vi "Kalman_Filter_Generator.vi"(8 "error in (no error)":errorcluster, 9 "Threshold":dbl, 10 "State Variance":dbl, 11 "Measurement Variance":dbl) -> (0 "error out":errorcluster, 3 "Kalman_Filter out":refnum<class "Kalman_Filter.lvclass">)   [LabVIEW 2021, in "Kalman_Filter.lvclass"]
uses:
  Kalman_Filter.lvclass
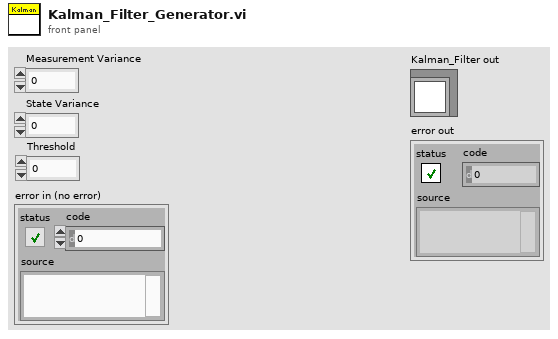
[diagram p1: front panel]
types:
  T1 = cluster{"State":dbl[][], "F state prop matrix":dbl[][], "H measure matrix":dbl[][], "P process cov":dbl[][], "R measure cov":dbl[][], "Q state cov":dbl[][], "T Sample":dbl, "New Measurement":dbl, "Measurement Variance":dbl, "State Variance":dbl, "Threshold":dbl, "Initialized":bool}
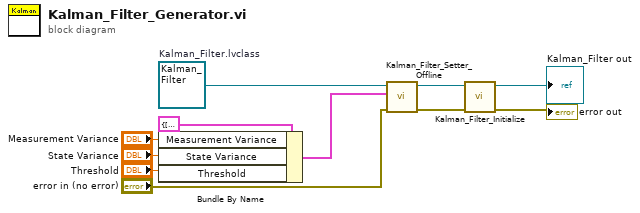
[diagram p0: block diagram]
diagram:
  w11 = refnum<class "Kalman_Filter.lvclass"> refnum  # Kalman_Filter.lvclass
  n1 = Bundle By Name(cluster=T1 {"State"=[], "F state prop matrix"=[], "H measure matrix"=[], "P process cov"=[], "R measure cov"=[], "Q state cov"=[], "T Sample"=0.0, "New Measurement"=0.0, "Measurement Variance"=0.0, "State Variance"=0.0, "Threshold"=0.0, "Initialized"=FALSE} ("KF"), "Measurement Variance"="Measurement Variance", "State Variance"="State Variance", "Threshold"="Threshold") -> (w9:T1)
  n2 = call-dynamic "Kalman_Filter_Setter_Offline.vi"("error in (no error)"="error in (no error)", "KF"=w9, "Kalman_Filter in"=w11) -> ("error out"=w8:errorcluster, "Kalman_Filter out"=w7:refnum<class "Kalman_Filter.lvclass">)  [unwired: 7 in]
  n3 = call-dynamic "Kalman_Filter_Initialize.vi"("error in (no error)"=w8, "Kalman_Filter in"=w7) -> ("error out"=→"error out":errorcluster, "Kalman_Filter out"=→"Kalman_Filter out":refnum<class "Kalman_Filter.lvclass">)  [unwired: 8 in]
